vi "Lidar Control Classical Controler.vi"(5 "Lidar Motor Control":T1={"Reset Encoder"=FALSE, "Motor Enable"=FALSE, "Choice of Control Type"=enum."Direct Voltage Control", "Choice of Oscillation"=enum."Oscillate Voltage", "Choice of Compensation"=enum."None", "Choice of Error"=enum."Gray Error", "Units of pi rad 18b (s-fxp-1)"={"Phi_B Set Point (pi rad)"=0.0, "Phi_A Set Point (pi rad)"=0.0, "Phi_Lidar Set Point (pi rad)"=0.0, "Phi_Lidar - Phi_A"=0.0, "Phi_mass-Phi_Lidar"=0.0, "Convert (enc) to (pi rad)"=0.0, "Oscillation Frequency (pi rad per 100KHz)"=0.0}, "Units of 18b (s-fxp-1) gain"={"Proportional Gain"=0.0, " Integral Gain"=0.0, "Oscillation Setpoint Amplitude"=0.0, "Gravity Compensation Gain"=0.0, "Phi_B Set Point (enc) pre-gain"=0.0, "Phi_B Set Point (pi rad) pre-gain"=0.0, "Phi_A Set Point (pi rad) pre-gain"=0.0, "Phi_Lidar Set Point (pi rad) pre-gain"=0.0, "Derivative Gain"=0.0, "Double Integral Gain"=0.0, "Second Derivative Gain"=0.0}, "Units of 20b s-fxp-5 Voltage"={"Oscillation Voltage Amplitude"=0.0, "Motor Voltage"=0.0}, "Units of encoder 32b uint"={"Phi_B Set Point (enc)"=0, "Lidar Encoder Cap"=0}, "Debug Args"=[FALSE, FALSE, FALSE, FALSE, FALSE, FALSE, FALSE, FALSE, FALSE, FALSE, FALSE, FALSE, FALSE, FALSE, FALSE, FALSE, FALSE, FALSE, FALSE, FALSE], "Units of 8b int gain exponents"={"Proportional Gain"=0, " Integral Gain"=0, "Oscillation Setpoint Amplitude"=0, "Gravity Compensation Gain"=0, "Phi_B Set Point (enc) pre-gain"=0, "Phi_B Set Point (pi rad) pre-gain"=0, "Phi_A Set Point (pi rad) pre-gain"=0, "Phi_Lidar Set Point (pi rad) pre-gain"=0, "Derivative Gain"=0, "Double Integral Gain"=0, "Second Derivative Gain"=0}, "6b (u-fxp-6)"={"Size of Integrator"=0.0, "Size of IIntigrator"=0.0, "Size of Differentiator"=0.0, "Size of DDifferentiator"=0.0}} {"Units of 20b s-fxp-5 Voltage"."Motor Voltage" format="%.17g"}) -> (1 "Motor Command":fxp<+/-,18,1> format="%.18g")   [LabVIEW 2010]
uses:
  [Debug] Global.vi
  Strict Lidar Motor Control Cluster.ctl
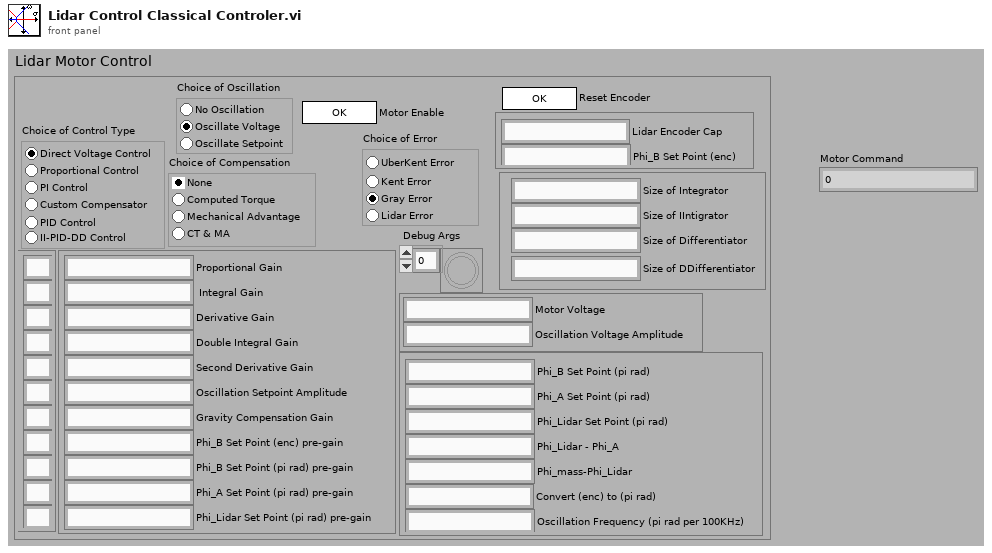
[diagram p1: front panel]
types:
  T1 = typedef "Strict Lidar Motor Control Cluster.ctl" = cluster{"Reset Encoder":bool, "Motor Enable":bool, "Choice of Control Type":enum32{"Direct Voltage Control", "Proportional Control", "PI Control", "Custom Compensator", "PID Control", "II-PID-DD Control"}, "Choice of Oscillation":enum32{"Oscillate Voltage", "Oscillate Setpoint", "No Oscillation"}, "Choice of Compensation":enum32{"None", "Computed Torque", "Mechanical Advantage", "CT & MA "}, "Choice of Error":enum32{"Gray Error", "Lidar Error", "Kent Error", "UberKent Error"}, "Units of pi rad 18b (s-fxp-1)":cluster{"Phi_B Set Point (pi rad)":fxp<+/-,18,1>, "Phi_A Set Point (pi rad)":fxp<+/-,18,1>, "Phi_Lidar Set Point (pi rad)":fxp<+/-,18,1>, "Phi_Lidar - Phi_A":fxp<+/-,18,1>, "Phi_mass-Phi_Lidar":fxp<+/-,18,1>, "Convert (enc) to (pi rad)":fxp<+/-,18,1>, "Oscillation Frequency (pi rad per 100KHz)":fxp<+/-,18,1>}, "Units of 18b (s-fxp-1) gain":cluster{"Proportional Gain":fxp<+/-,18,1>, " Integral Gain":fxp<+/-,18,1>, "Oscillation Setpoint Amplitude":fxp<+/-,18,1>, "Gravity Compensation Gain":fxp<+/-,18,1>, "Phi_B Set Point (enc) pre-gain":fxp<+/-,18,1>, "Phi_B Set Point (pi rad) pre-gain":fxp<+/-,18,1>, "Phi_A Set Point (pi rad) pre-gain":fxp<+/-,18,1>, "Phi_Lidar Set Point (pi rad) pre-gain":fxp<+/-,18,1>, "Derivative Gain":fxp<+/-,18,1>, "Double Integral Gain":fxp<+/-,18,1>, "Second Derivative Gain":fxp<+/-,18,1>}, "Units of 20b s-fxp-5 Voltage":cluster{"Oscillation Voltage Amplitude":fxp<+/-,20,5>, "Motor Voltage":fxp<+/-,20,5>}, "Units of encoder 32b uint":cluster{"Phi_B Set Point (enc)":i32, "Lidar Encoder Cap":i32}, "Debug Args":bool[], "Units of 8b int gain exponents":cluster{"Proportional Gain":i8, " Integral Gain":i8, "Oscillation Setpoint Amplitude":i8, "Gravity Compensation Gain":i8, "Phi_B Set Point (enc) pre-gain":i8, "Phi_B Set Point (pi rad) pre-gain":i8, "Phi_A Set Point (pi rad) pre-gain":i8, "Phi_Lidar Set Point (pi rad) pre-gain":i8, "Derivative Gain":i8, "Double Integral Gain":i8, "Second Derivative Gain":i8}, "6b (u-fxp-6)":cluster{"Size of Integrator":fxp<+,6,6>, "Size of IIntigrator":fxp<+,6,6>, "Size of Differentiator":fxp<+,6,6>, "Size of DDifferentiator":fxp<+,6,6>}}
  T2 = enum32{"Direct Voltage Control", "Proportional Control", "PI Control", "Custom Compensator", "PID Control", "II-PID-DD Control"}
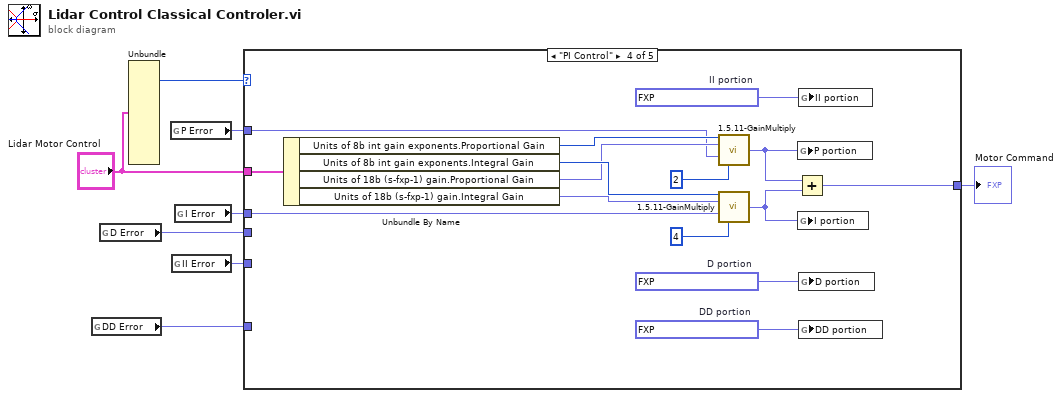
[diagram p0: block diagram]
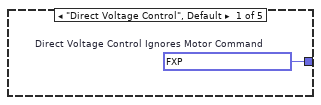
[diagram p2: hidden frame]
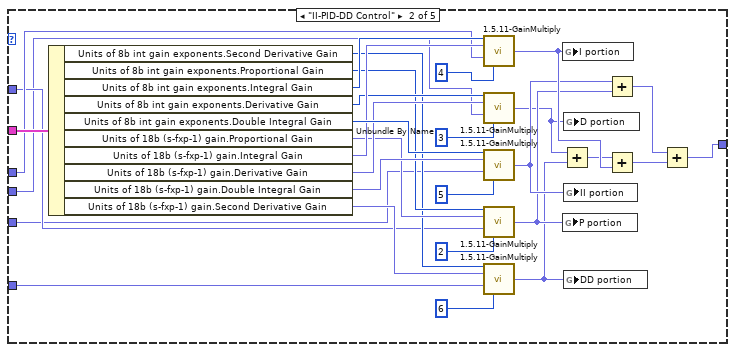
[diagram p3: hidden frame]
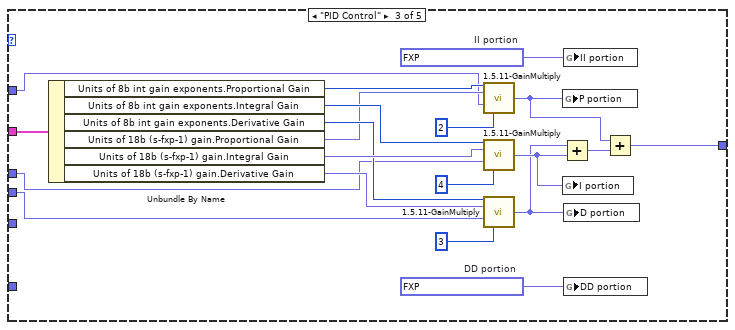
[diagram p4: hidden frame]
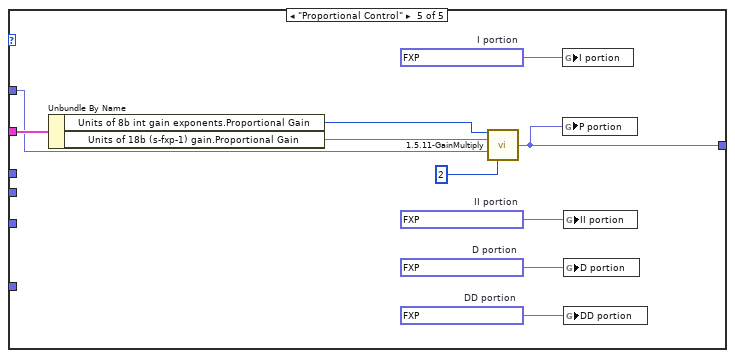
[diagram p5: hidden frame]
diagram:
  n1 = global read "[Debug] Global.vi" "DD Error"() -> (w3:fxp<+/-,18,1>)
  n2 = global read "[Debug] Global.vi" "D Error"() -> (w2:fxp<+/-,18,1>)
  n3 = Unbundle("Lidar Motor Control") -> ("Choice of Control Type"=w6:T2)  [unwired: 12 out]
  n4 = global read "[Debug] Global.vi" "P Error"() -> (w5:fxp<+/-,18,1>)
  n5 = global read "[Debug] Global.vi" "II Error"() -> (w1:fxp<+/-,18,1>)
  n6 = global read "[Debug] Global.vi" "I Error"() -> (w4:fxp<+/-,18,1>)
  n7 = case shown="\"PI Control\"" w6 {
    tunnel: [w9 w39 w59 w74 w77] -> w8
    tunnel: "Lidar Motor Control" -> [_ w27 w50 w68 w82]
    tunnel: w5 -> [_ w13 w45 w65 w75]
    tunnel: w4 -> [_ w14 w46 w66 _]
    tunnel: w3 -> [_ w12 _ _ _]
    tunnel: w2 -> [_ w11 w44 _ _]
    tunnel: w1 -> [_ w10 _ _ _]
    frame "Direct Voltage Control", Default {
      w9 = fxp<+/-,18,1> -1.0  # Direct Voltage Control Ignores Motor Command
    }
    frame "II-PID-DD Control" {
      n8 = Unbundle By Name(w27) -> ("Units of 8b int gain exponents.Second Derivative Gain"=w18:i8, "Units of 8b int gain exponents.Proportional Gain"=w28:i8, "Units of 8b int gain exponents.Integral Gain"=w32:i8, "Units of 8b int gain exponents.Derivative Gain"=w30:i8, "Units of 8b int gain exponents.Double Integral Gain"=w34:i8, "Units of 18b (s-fxp-1) gain.Proportional Gain"=w29:fxp<+/-,18,1>, "Units of 18b (s-fxp-1) gain.Integral Gain"=w33:fxp<+/-,18,1>, "Units of 18b (s-fxp-1) gain.Derivative Gain"=w31:fxp<+/-,18,1>, "Units of 18b (s-fxp-1) gain.Double Integral Gain"=w35:fxp<+/-,18,1>, "Units of 18b (s-fxp-1) gain.Second Derivative Gain"=w19:fxp<+/-,18,1>)
      n9 = call "1.5.11-GainMultiply.vi"("Gain Exponent"=w32, "Gain"=w33, "Input"=w14, "Unique 8b identifier"=u8 4) -> ("Output"=w26:fxp<+/-,18,1>)  [unwired: 9 in, 2 out]
      n10 = call "1.5.11-GainMultiply.vi"("Gain Exponent"=w30, "Gain"=w31, "Input"=w11, "Unique 8b identifier"=u8 3) -> ("Output"=w17:fxp<+/-,18,1>)  [unwired: 9 in, 2 out]
      n11 = call "1.5.11-GainMultiply.vi"("Gain Exponent"=w34, "Gain"=w35, "Input"=w10, "Unique 8b identifier"=u8 5) -> ("Output"=w25:fxp<+/-,18,1>)  [unwired: 9 in, 2 out]
      n12 = call "1.5.11-GainMultiply.vi"("Gain Exponent"=w28, "Gain"=w29, "Input"=w13, "Unique 8b identifier"=u8 2) -> ("Output"=w24:fxp<+/-,18,1>)  [unwired: 9 in, 2 out]
      n13 = call "1.5.11-GainMultiply.vi"("Gain Exponent"=w18, "Gain"=w19, "Input"=w12, "Unique 8b identifier"=u8 6) -> ("Output"=w15:fxp<+/-,18,1>)  [unwired: 9 in, 2 out]
      n14 = Add(x=w17, y=w15) -> (x+y=w16:fxp<+/-,18,1>)
      n15 = global write "[Debug] Global.vi" "I portion"(w26) -> ()
      n16 = global write "[Debug] Global.vi" "P portion"(w24) -> ()
      n17 = global write "[Debug] Global.vi" "D portion"(w17) -> ()
      n18 = global write "[Debug] Global.vi" "II portion"(w25) -> ()
      n19 = global write "[Debug] Global.vi" "DD portion"(w15) -> ()
      n20 = Add(x=w25, y=w24) -> (x+y=w22:fxp<+/-,18,1>)
      n21 = Add(x=w16, y=w26) -> (x+y=w23:fxp<+/-,18,1>)
      n22 = Add(x=w22, y=w23) -> (x+y=w39:fxp<+/-,18,1>)
    }
    frame "PID Control" {
      w40 = fxp<+/-,18,1> 0.0  # II portion
      w43 = fxp<+/-,18,1> 0.0  # DD portion
      n23 = Unbundle By Name(w50) -> ("Units of 8b int gain exponents.Proportional Gain"=w51:i8, "Units of 8b int gain exponents.Integral Gain"=w55:i8, "Units of 8b int gain exponents.Derivative Gain"=w53:i8, "Units of 18b (s-fxp-1) gain.Proportional Gain"=w52:fxp<+/-,18,1>, "Units of 18b (s-fxp-1) gain.Integral Gain"=w56:fxp<+/-,18,1>, "Units of 18b (s-fxp-1) gain.Derivative Gain"=w54:fxp<+/-,18,1>)
      n24 = call "1.5.11-GainMultiply.vi"("Gain Exponent"=w51, "Gain"=w52, "Input"=w45, "Unique 8b identifier"=u8 2) -> ("Output"=w42:fxp<+/-,18,1>)  [unwired: 9 in, 2 out]
      n25 = call "1.5.11-GainMultiply.vi"("Gain Exponent"=w55, "Gain"=w56, "Input"=w46, "Unique 8b identifier"=u8 4) -> ("Output"=w49:fxp<+/-,18,1>)  [unwired: 9 in, 2 out]
      n26 = call "1.5.11-GainMultiply.vi"("Gain Exponent"=w53, "Gain"=w54, "Input"=w44, "Unique 8b identifier"=u8 3) -> ("Output"=w41:fxp<+/-,18,1>)  [unwired: 9 in, 2 out]
      n27 = Add(x=w41, y=w49) -> (x+y=w48:fxp<+/-,18,1>)
      n28 = global write "[Debug] Global.vi" "P portion"(w42) -> ()
      n29 = global write "[Debug] Global.vi" "I portion"(w49) -> ()
      n30 = global write "[Debug] Global.vi" "II portion"(w40) -> ()
      n31 = global write "[Debug] Global.vi" "D portion"(w41) -> ()
      n32 = global write "[Debug] Global.vi" "DD portion"(w43) -> ()
      n33 = Add(x=w42, y=w48) -> (x+y=w59:fxp<+/-,18,1>)
    }
    frame "PI Control" {
      w61 = fxp<+/-,18,1> 0.0  # D portion
      w62 = fxp<+/-,18,1> 0.0  # II portion
      w64 = fxp<+/-,18,1> 0.0  # DD portion
      n34 = Unbundle By Name(w68) -> ("Units of 8b int gain exponents.Proportional Gain"=w69:i8, "Units of 8b int gain exponents.Integral Gain"=w71:i8, "Units of 18b (s-fxp-1) gain.Proportional Gain"=w70:fxp<+/-,18,1>, "Units of 18b (s-fxp-1) gain.Integral Gain"=w72:fxp<+/-,18,1>)
      n35 = call "1.5.11-GainMultiply.vi"("Gain Exponent"=w69, "Gain"=w70, "Input"=w65, "Unique 8b identifier"=u8 2) -> ("Output"=w63:fxp<+/-,18,1>)  [unwired: 9 in, 2 out]
      n36 = call "1.5.11-GainMultiply.vi"("Gain Exponent"=w71, "Gain"=w72, "Input"=w66, "Unique 8b identifier"=u8 4) -> ("Output"=w60:fxp<+/-,18,1>)  [unwired: 9 in, 2 out]
      n37 = Add(x=w63, y=w60) -> (x+y=w74:fxp<+/-,18,1>)
      n38 = global write "[Debug] Global.vi" "P portion"(w63) -> ()
      n39 = global write "[Debug] Global.vi" "I portion"(w60) -> ()
      n40 = global write "[Debug] Global.vi" "II portion"(w62) -> ()
      n41 = global write "[Debug] Global.vi" "D portion"(w61) -> ()
      n42 = global write "[Debug] Global.vi" "DD portion"(w64) -> ()
    }
    frame "Proportional Control" {
      w76 = fxp<+/-,18,1> 0.0  # I portion
      w78 = fxp<+/-,18,1> 0.0  # D portion
      w79 = fxp<+/-,18,1> 0.0  # II portion
      w80 = fxp<+/-,18,1> 0.0  # DD portion
      n43 = Unbundle By Name(w82) -> ("Units of 8b int gain exponents.Proportional Gain"=w83:i8, "Units of 18b (s-fxp-1) gain.Proportional Gain"=w84:fxp<+/-,18,1>)
      n44 = call "1.5.11-GainMultiply.vi"("Gain Exponent"=w83, "Gain"=w84, "Input"=w75, "Unique 8b identifier"=u8 2) -> ("Output"=w77:fxp<+/-,18,1>)  [unwired: 9 in, 2 out]
      n45 = global write "[Debug] Global.vi" "I portion"(w76) -> ()
      n46 = global write "[Debug] Global.vi" "P portion"(w77) -> ()
      n47 = global write "[Debug] Global.vi" "II portion"(w79) -> ()
      n48 = global write "[Debug] Global.vi" "D portion"(w78) -> ()
      n49 = global write "[Debug] Global.vi" "DD portion"(w80) -> ()
    }
  }
  "Motor Command" <- w8
